vi "CRYStep Read.vi"(6 "Category Name":string="stimulus.txt", 7 "error in":errorcluster, 8 "Proper VI No":i32, 9 "Step File Path":path=path "C:/") -> (0 "status":bool, 2 "selected path":path, 3 "Flatten Step":string)   [LabVIEW 2013]
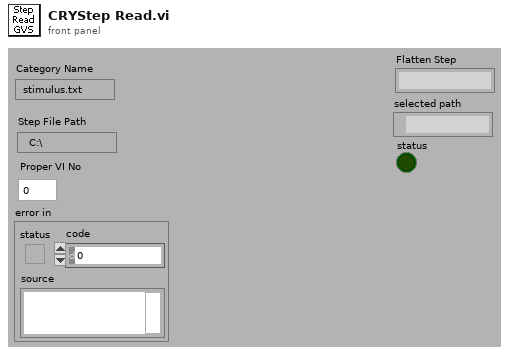
[diagram p1: front panel]
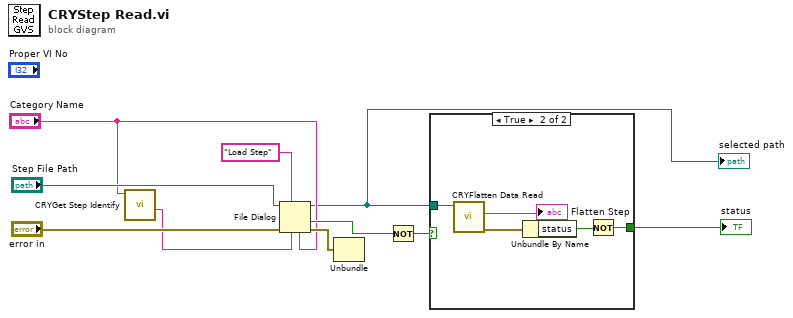
[diagram p0: block diagram]
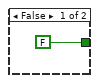
[diagram p2: hidden frame]
diagram:
  n1 = call "CRYGet Step Identify.vi"("Category Name In"="Category Name") -> ("Identfier(*.)"=w4:string)  [unwired: 3 in, 7 out]
  n2 = File Dialog(4:"Category Name", 6:w4, 7:"Load Step", 8:"error in", 11:"Step File Path") -> (0:w6:errorcluster, 1:w7:bool, 3:w1:path)  [unwired: 3 out]
  "selected path" <- w1
  n3 = Unbundle(w6) -> ()  [unwired: 3 out]
  n4 = Not(x=w7) -> (.not. x?=w5:bool)
  n5 = case shown="True" w5 {
    tunnel: w1 -> [_ w14]
    tunnel: [FALSE ("status") w15] -> w2
    frame False {
    }
    frame True {
      n6 = call "CRYFlatten Data Read.vi"("Path In"=w14) -> ("error out"=w13:errorcluster, "Flatten Data Out"=→"Flatten Step":string)  [unwired: 6 in, 1 out]
      n7 = Unbundle By Name(w13) -> ("status"=w16:bool)
      n8 = Not(x=w16) -> (.not. x?=w15:bool)
    }
  }
  "status" <- w2
